vi "EXAMPLE - Dynamic Shared Variables.vi"() -> ()   [LabVIEW 2018, in "Dynamic Shared Variables.lvlib"]
uses:
  Dynamic Shared Variables.lvlib
  Tag VIs/Tag FGV Operation Enum.ctl
panel:
  in  "stop":bool
  out "error out":errorcluster
  # "INSTRUCTIONS:\n1. Run this VI\n2. Open Distributed Systems Manager and  select View->Refresh (or press F5).\n3. In DSM, observe that there should be a Pfizer FAST process with date/timestamp. Under the process there should be a mytag DBL shared variable.\n4. Press the STOP button.\n5. In DSM, press Refresh (or F5), observe that the Pfizer_FAST process disappears."
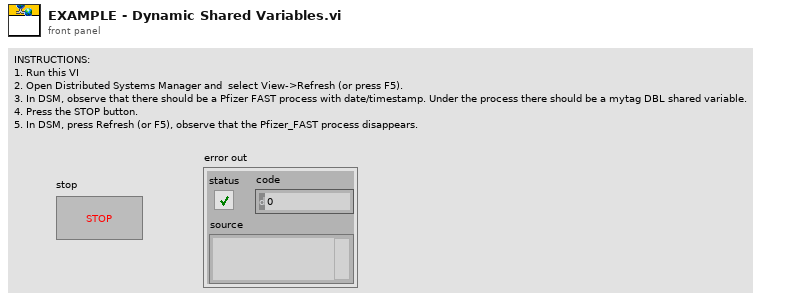
[diagram p1: front panel]
types:
  T1 = enum32{"u32BitField", "bool", "double", "string", "int8", "uint8", "int16", "uint16", "int32", "uint32", "int64", "uint64", "single", "double waveform", "int16 waveform", "array of boolean", "array of int8", "array of uint8", "array of int16", "array of uint16", "array of int32", "array of uint32", "array of int64", "array of uint64", "array of single", "array of double", "array of double waveform", "array of int16 waveform", "array of string", "variant", "timestamp", "fixed point", "custom"}
  T2 = typedef "Tag FGV Operation Enum.ctl" = enum16{"Init", "Set Notification Queue", "Create Tag", "Commit", "Write Tag (Numeric)", "Write Tag (Boolean)", "Read All Tags", "Read One Tag", "Delete Tag Category", "Set Alarm Parameters (Numeric)", "Set Alarm Parameters (Boolean)", "Enable All Alarms", "Disable All Alarms", "Delete All Tags", "Read Alarms", "Ack Alarm", "Read Alarm Parameters (Numeric)", "Read Alarm Parameters (Boolean)"}
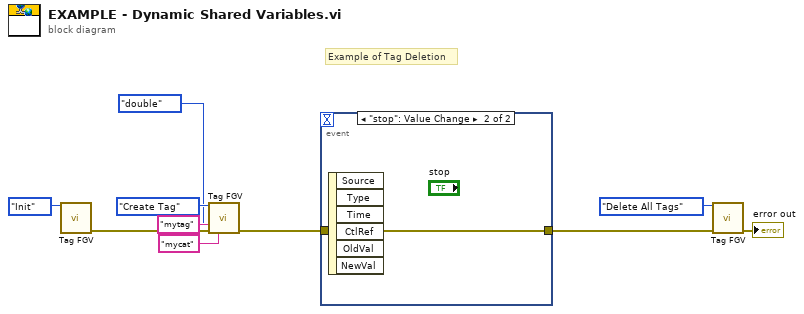
[diagram p0: block diagram]
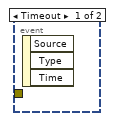
[diagram p2: hidden frame]
diagram:
  # "Example of Tag Deletion"
  n1 = call "Tag FGV.vi"("Operation"=Tag_FGV_Operation_Enum."Init") -> ("error out"=w5:errorcluster)  [unwired: 7 in, 7 out]
  n2 = call "Tag FGV.vi"("Operation"=Tag_FGV_Operation_Enum."Create Tag", "Tag Name"="mytag", "Data"=T1."double" ("data type"), "error in (no error)"=w5, "Tag Category"="mycat") -> ("error out"=w4:errorcluster)  [unwired: 3 in, 7 out]
  n3 = event shown="[1] \"stop\": Value Change" {
    selector: _ -> [_ _]
    dyn-events: _ -> [_ _]
    timeout: _ -> [_ _]
    tunnel: [_ w11] -> w7
    tunnel: w4 -> [_ w11]
    event Timeout {
      n4 = event-data() -> ()  [unwired: 1 in, 3 out]
    }
    event "stop": Value Change {
      n5 = event-data() -> ()  [unwired: 1 in, 6 out]
    }
  }
  n6 = call "Tag FGV.vi"("Operation"=Tag_FGV_Operation_Enum."Delete All Tags", "error in (no error)"=w7) -> ("error out"=→"error out":errorcluster)  [unwired: 6 in, 7 out]
